vi "Receiver_Example - 2 Channels.vi"() -> ()   [LabVIEW 2022 SP3]
panel:
  out "Constellation Map":cluster{"Constellation":cdb[]}[](graph)
  in  "Tab Control":enum32{"USRP Parameters", "Rx Info", "BER"}(tab)
  in  "USRP ControledParameters":T1={"Active Antenna"="RX2", "Gain (dB)"=10.0, "Carrier Frequency"=2400000000.0, "IQ Rate"=2000000.0, "Active channels"="0,1"} {"IQ Rate" format="%#_6p"; "Carrier Frequency" format="%#_6p"; "Gain (dB)" format="%#_6f"}
  in  "Device selection":refnum<k15>="RIO0"
  in  "Trigger level":dbl=0.005 format="%f"
  out "CH0":T2
  out "CH1":T2
  out "SIG valid? - CH1":bool
  out "SIG valid? - CH0":bool
  out "Frequency offset - CH1":dbl
  out "Frequency offset - CH0":dbl
  out "Coerced Parameters":T3={"IQ Rate"=100000.0, "Carrier  Freq."=100000.0, "Gain"=0.0} {"Gain" format="%#_6f"; "Carrier  Freq." format="%#_6p"; "IQ Rate" format="%#_6p"}
  out "Error out":errorcluster
  out "Acc. BER - CH1":dbl format="%#_4g"
  in  "Refresh Button":bool
  in  "Record BER":bool
  in  "Expected message - CH0":string="Hello World! aaaaaaaaaaaaaaaaaaaaaa\nHello World! aaaaaaaaaaaaaaaaaaaaaa\nHello World! aaaaaaaaaaaaaaaaaaaaaa\nHello World! aaaaaaaaaaaaaaaaaaaaaa"
  in  "Expected message - CH1":string="Hola Mundo! bbbbbbbbbbbbbbbbbbbbbbb\nHola Mundo! bbbbbbbbbbbbbbbbbbbbbbb\nHola Mundo! bbbbbbbbbbbbbbbbbbbbbbb\nHola Mundo! bbbbbbbbbbbbbbbbbbbbbbb"
  out "Acum. Err - CH0":dbl
  out "Acum. Err - CH1":dbl
  out "No. Bits - CH0":dbl
  out "No. Bits - CH1":dbl
  out "Inst. BER - CH0":dbl format="%#_4g"
  out "Inst. BER - CH1":dbl format="%#_4g"
  out "Acc. BER - CH0":dbl format="%#_4g"
  in  "Decode SC? - CH1":bool=TRUE
  in  "Decode SC? - CH0":bool
  in  "error in (no error)":errorcluster
  out "Decoded message - CH1":string
  out "Decoded message - CH0":string
  # "OFDM Superposition Coded Receiver"
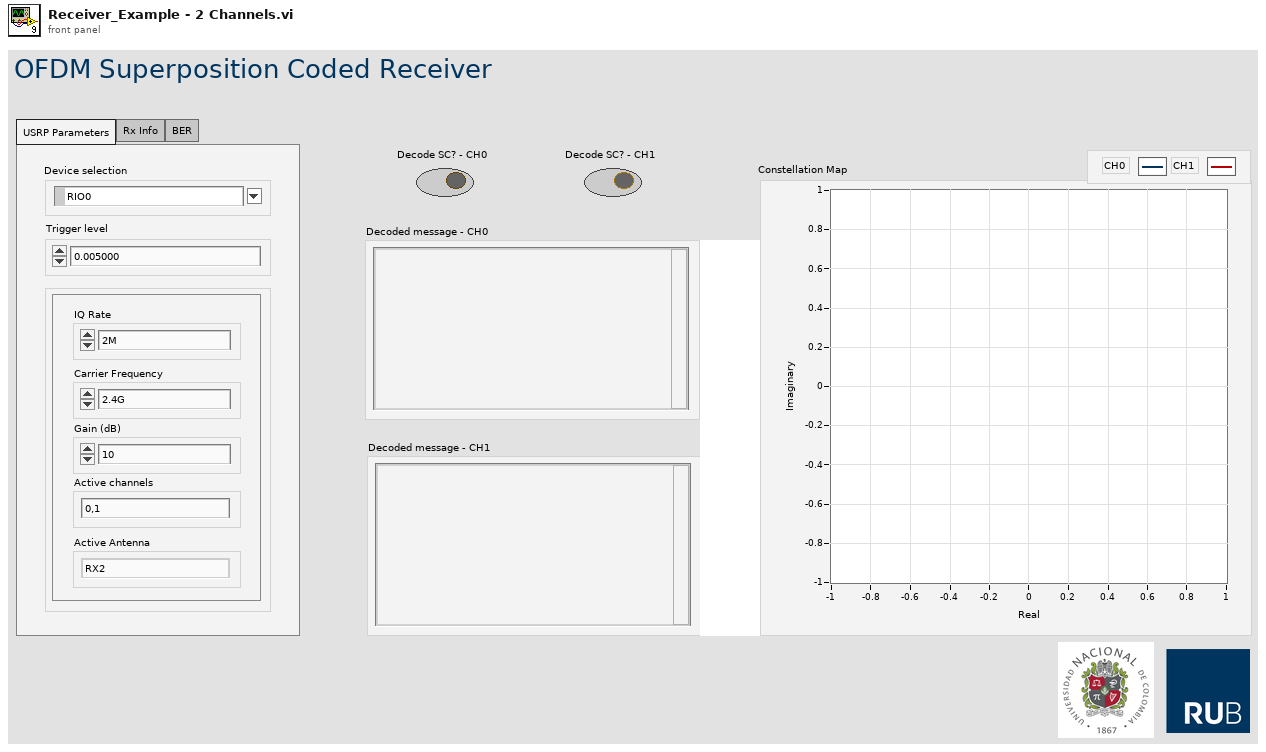
[diagram p1: front panel]
types:
  T1 = cluster{"Active Antenna":string, "Gain (dB)":dbl, "Carrier Frequency":dbl, "IQ Rate":dbl, "Active channels":string}
  T2 = cluster{"Modulation type":enum16{"QPSK(4QAM)", "64QAM", "16QAM", "BPSK"}, "BCC rate (k/n)":enum16{"1/2", "2/3", "3/4"}}
  T3 = cluster{"IQ Rate":dbl, "Carrier  Freq.":dbl, "Gain":dbl}
  T4 = cluster{"coerced IQ rate":dbl, "coerced carrier frequency":dbl, "coerced gain":dbl}
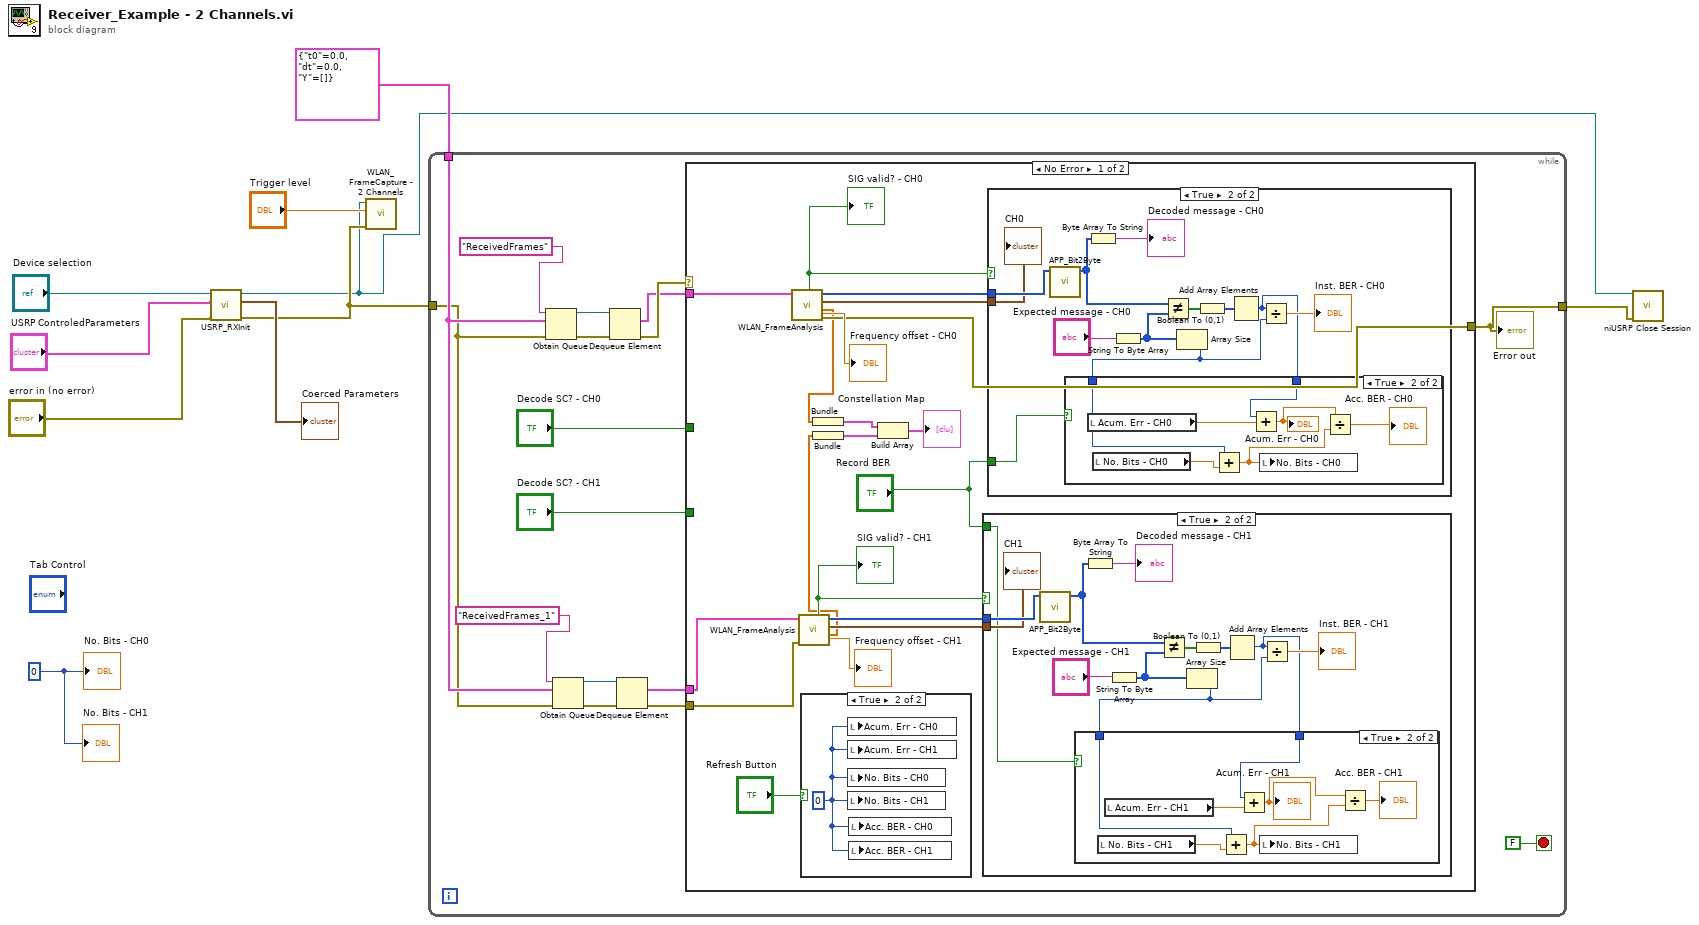
[diagram p0: block diagram]
diagram:
  w1 = 0
  n1 = call "USRP_RXInit.vi"("device names"="Device selection", "USRP ControledParameters"="USRP ControledParameters", "error in (no error)"="error in (no error)") -> ("session handle out"=w4:refnum<k15>, "USRP CoercedParamters"=→"Coerced Parameters":T4, "error out"=w8:errorcluster)  [unwired: 5 in]
  n2 = call "WLAN_FrameCapture - 2 Channels.vi"("error in (no error)"=w8, "Trigger level"="Trigger level", "session handle"=w4) -> ()  [unwired: 8 in]
  n3 = while {
    tunnel: w8 -> [w15]
    tunnel: cluster{"t0":dbl, "dt":dbl, "Y":cdb[]} {"t0"=0.0, "dt"=0.0, "Y"=[]} ("data") -> [w16]
    tunnel: [w21] -> w5
    stop <- FALSE stop-if-true
    n4 = Obtain Queue(name (unnamed)="ReceivedFrames", element data type=w16, error in (no error)=w15) -> (queue out=w26:refnum<queue>, error out=w23:errorcluster)  [unwired: 2 in, 1 out]
    n5 = Obtain Queue(name (unnamed)="ReceivedFrames_1", element data type=w16, error in (no error)=w15) -> (queue out=w19:refnum<queue>, error out=w18:errorcluster)  [unwired: 2 in, 1 out]
    n6 = Dequeue Element(queue=w26, error in (no error)=w23) -> (element=w24:cluster{"t0":dbl, "dt":dbl, "Y":cdb[]}, error out=w25:errorcluster)  [unwired: 1 in, 2 out]
    n7 = Dequeue Element(queue=w19, error in (no error)=w18) -> (element=w12:cluster{"t0":dbl, "dt":dbl, "Y":cdb[]}, error out=w13:errorcluster)  [unwired: 1 in, 2 out]
    n8 = case shown="No Error" w25 {
      selector: w25 -> [_ w85]
      tunnel: w24 -> [w40 _]
      tunnel: [w41 w85] -> w21
      tunnel: "Decode SC? - CH0" -> [_ _]
      tunnel: "Decode SC? - CH1" -> [_ _]
      tunnel: w13 -> [w35 _]
      tunnel: w12 -> [w34 _]
      frame No Error {
        n9 = call "WLAN_FrameAnalysis.vi"("input cluster"=w40) -> ("error out"=w41:errorcluster, "Constellation"=w33:cdb[], "Modulation parameter"=w42:T2, "output bits"=w43:i8[], "Frequency offset"=→"Frequency offset - CH0":dbl, "SIG valid?"=w44:bool)  [unwired: 4 in, 1 out]
        "SIG valid? - CH0" <- w44
        n10 = call "WLAN_FrameAnalysis.vi"("error in (no error)"=w35, "input cluster"=w34) -> ("Constellation"=w32:cdb[], "Modulation parameter"=w36:T2, "output bits"=w37:i8[], "Frequency offset"=→"Frequency offset - CH1":dbl, "SIG valid?"=w38:bool)  [unwired: 3 in, 2 out]
        "SIG valid? - CH1" <- w38
        n11 = case shown="True" "Refresh Button" {
          frame False {
          }
          frame True {
            w46 = 0
            n12 = local write "Acum. Err - CH0"(w46) -> ()
            n13 = local write "Acum. Err - CH1"(w46) -> ()
            n14 = local write "No. Bits - CH0"(w46) -> ()
            n15 = local write "No. Bits - CH1"(w46) -> ()
            n16 = local write "Acc. BER - CH0"(w46) -> ()
            n17 = local write "Acc. BER - CH1"(w46) -> ()
          }
        }
        n18 = Bundle("Constellation"=w33) -> (w29:cluster{"Constellation":cdb[]})  [unwired: 1 in]
        n19 = Bundle("Constellation"=w32) -> (w30:cluster{"Constellation":cdb[]})  [unwired: 1 in]
        n20 = Build Array(w29, w30) -> (→"Constellation Map":cluster{"Constellation":cdb[]}[])
        n21 = case shown="True" w38 {
          tunnel: w37 -> [_ w58]
          tunnel: w36 -> [_ w57]
          tunnel: "Record BER" -> [_ w51]
          frame False {
          }
          frame True {
            n22 = call "APP_Bit2Byte.vi"("input bit stream"=w58) -> ("output byte stream"=w53:u8[])  [unwired: 10 in]
            n23 = Byte Array To String(unsigned byte array=w53) -> (string=→"Decoded message - CH1":string)
            n24 = String To Byte Array(string="Expected message - CH1") -> (unsigned byte array=w49:u8[])
            n25 = Not Equal?(x=w53, y=w49) -> (x != y?=w54:bool[])
            n26 = Array Size(array=w49) -> (size(s)=w48:i32)
            n27 = Boolean To (0,1)(Boolean=w54) -> (0, 1=w55:i16[])
            n28 = Add Array Elements(numeric array=w55) -> (sum=w47:i16)
            n29 = case shown="True" w51 {
              tunnel: w48 -> [_ w64]
              tunnel: w47 -> [_ w62]
              frame False {
              }
              frame True {
                n30 = local read "No. Bits - CH1"() -> (w65:dbl)
                n31 = local read "Acum. Err - CH1"() -> (w63:dbl)
                n32 = Add(x=w64, y=w65) -> (x+y=w61:dbl)
                n33 = Add(x=w62, y=w63) -> (x+y=w60:dbl)
                "Acum. Err - CH1" <- w60
                n34 = local write "No. Bits - CH1"(w61) -> ()
                n35 = Divide(x=w60, y=w61) -> (x/y=→"Acc. BER - CH1":dbl)
              }
            }
            n36 = Divide(x=w47, y=w48) -> (x/y=→"Inst. BER - CH1":dbl)
            "CH1" <- w57
          }
        }
        n37 = case shown="True" w44 {
          tunnel: w43 -> [_ w77]
          tunnel: w42 -> [_ w75]
          tunnel: "Record BER" -> [_ w70]
          frame False {
          }
          frame True {
            n38 = call "APP_Bit2Byte.vi"("input bit stream"=w77) -> ("output byte stream"=w72:u8[])  [unwired: 10 in]
            n39 = Byte Array To String(unsigned byte array=w72) -> (string=→"Decoded message - CH0":string)
            n40 = String To Byte Array(string="Expected message - CH0") -> (unsigned byte array=w69:u8[])
            n41 = Not Equal?(x=w72, y=w69) -> (x != y?=w73:bool[])
            n42 = Array Size(array=w69) -> (size(s)=w67:i32)
            n43 = Boolean To (0,1)(Boolean=w73) -> (0, 1=w74:i16[])
            n44 = Add Array Elements(numeric array=w74) -> (sum=w66:i16)
            n45 = case shown="True" w70 {
              tunnel: w67 -> [_ w83]
              tunnel: w66 -> [_ w81]
              frame False {
              }
              frame True {
                n46 = local read "Acum. Err - CH0"() -> (w82:dbl)
                n47 = local read "No. Bits - CH0"() -> (w84:dbl)
                n48 = Add(x=w83, y=w84) -> (x+y=w80:dbl)
                n49 = Add(x=w81, y=w82) -> (x+y=w79:dbl)
                "Acum. Err - CH0" <- w79
                n50 = local write "No. Bits - CH0"(w80) -> ()
                n51 = Divide(x=w79, y=w80) -> (x/y=→"Acc. BER - CH0":dbl)
              }
            }
            n52 = Divide(x=w66, y=w67) -> (x/y=→"Inst. BER - CH0":dbl)
            "CH0" <- w75
          }
        }
      }
      frame Error {
      }
    }
    "Error out" <- w21
  }
  n53 = call <instrlib>:"niUSRP Close Session.vi"("session handle"=w4, "error in (no error)"=w5) -> ()  [unwired: 13 in, 1 out]
  "No. Bits - CH0" <- w1
  "No. Bits - CH1" <- w1
